vi "Download Waveform.vi"(0 "RFSG handle":refnum<k15>, 5 "Waveform In":T1={"Waveform Name"="Wfm", "Waveform"={"x0"=0.0, "dx"=0.0, "y"=[]}, "Signal Bandwidth (Hz)"=0.0, "PAPR (dB)"=0.0, "Burst Length (s)"=0.0, "Sample Rate"=0.0, "Burst Start Locations"=[], "Burst Stop Locations"=[], "Idle Duration Present?"=FALSE, "Runtime Scaling"=0.0, "Script"=""} {"Runtime Scaling" format="%#_6p"; "Sample Rate" format="%#_6p"; "Burst Length (s)" format="%#_6p"; "PAPR (dB)" format="%.2f"; "Signal Bandwidth (Hz)" format="%.2f"; "Waveform"."y" format="%.2f"; "Waveform"."dx" format="%^.2e"; "Waveform"."x0" format="%^.2e"}, 11 "error in (no error)":errorcluster) -> (4 "RFSG handle out":refnum<k15>, 15 "error out":errorcluster)   [LabVIEW 2016, in "SG.lvlib"]
uses:
  SG.lvlib
  Typedefs/Waveform.ctl
  <instrlib>/niRFSG/niRFSG.llb/niRFSG Write Arb Waveform (Complex Input SGL).vi
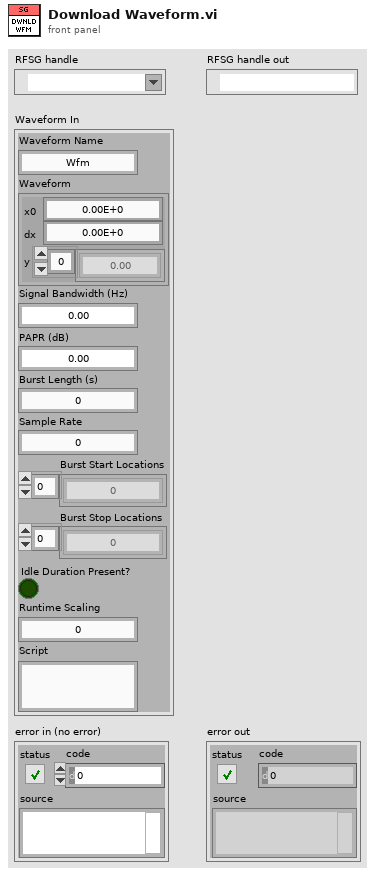
[diagram p1: front panel]
types:
  T1 = typedef "SG.lvlib/Waveform.ctl" = cluster{"Waveform Name":string, "Waveform":cluster{"x0":dbl, "dx":dbl, "y":csg[]}, "Signal Bandwidth (Hz)":dbl, "PAPR (dB)":dbl, "Burst Length (s)":dbl, "Sample Rate":dbl, "Burst Start Locations":i32[], "Burst Stop Locations":i32[], "Idle Duration Present?":bool, "Runtime Scaling":dbl, "Script":string}
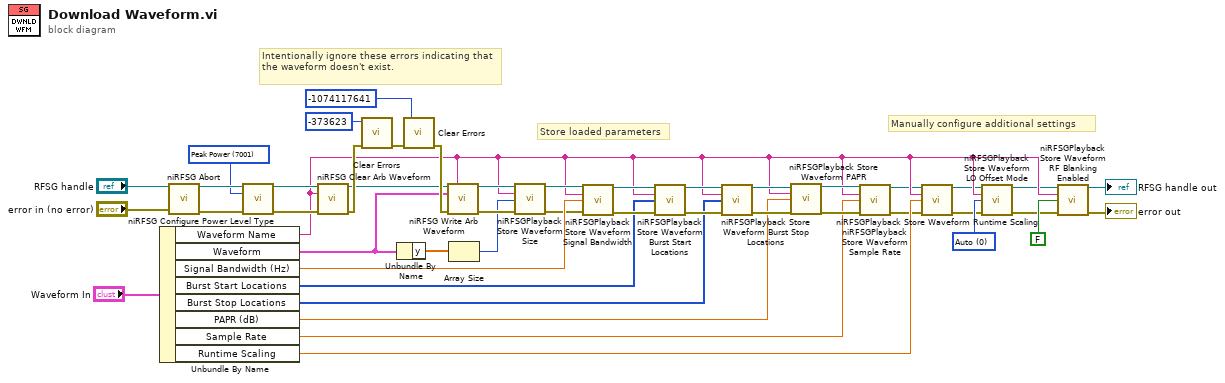
[diagram p0: block diagram]
diagram:
  w16 = 7001 items=["Average Power"=7000, "Peak Power"=7001] ("power level type")
  w32 = 0 items=["Auto", "No Offset", "Disabled"] ("LO offset mode")
  # "Manually configure additional settings"
  # "Store loaded parameters"
  # "Intentionally ignore these errors indicating that the waveform doesn't exist."
  n1 = Unbundle By Name("Waveform In") -> ("Waveform Name"=w7:string, "Waveform"=w10:cluster{"x0":dbl, "dx":dbl, "y":csg[]}, "Signal Bandwidth (Hz)"=w30:dbl, "Burst Start Locations"=w27:i32[], "Burst Stop Locations"=w24:i32[], "PAPR (dB)"=w23:dbl, "Sample Rate"=w19:dbl, "Runtime Scaling"=w14:dbl)
  n2 = call <instrlib>:"niRFSG Abort.vi"("instrument handle"="RFSG handle", "error in"="error in (no error)") -> ("instrument handle out"=w18:refnum<k15>, "error out"=w41:errorcluster)  [unwired: 12 in]
  n3 = call <instrlib>:"niRFSG Configure Power Level Type.vi"("instrument handle"=w18, "power level type"=w16, "error in"=w41) -> ("instrument handle out"=w17:refnum<k15>, "error out"=w36:errorcluster)  [unwired: 11 in]
  n4 = call <instrlib>:"niRFSG Clear Arb Waveform.vi"("instrument handle"=w17, "name"=w7, "error in"=w36) -> ("instrument handle out"=w31:refnum<k15>, "error out"=w40:errorcluster)  [unwired: 11 in]
  n5 = call <vilib>:"Clear Errors.vi"("error in (no error)"=w40, "specific error code to clear (0: all)"=-373623) -> ("error out"=w44:errorcluster)  [unwired: 4 in, 1 out]
  n6 = Unbundle By Name(w10) -> ("y"=w9:csg[])
  n7 = call <vilib>:"Clear Errors.vi"("error in (no error)"=w44, "specific error code to clear (0: all)"=-1074117641) -> ("error out"=w43:errorcluster)  [unwired: 4 in, 1 out]
  n8 = call-poly <instrlib>:"niRFSG Write Arb Waveform.vi"("instrument handle"=w31, "name"=w7, "IQ waveform"=w10, "error in"=w43) -> ("instrument handle out"=w12:refnum<k15>, "error out"=w15:errorcluster)  [unwired: 10 in]
  n9 = Array Size(array=w9) -> (size(s)=w8:i32)
  n10 = call <instrlib>:"niRFSGPlayback Store Waveform Size.vi"("instrument handle in"=w12, "waveform name"=w7, "waveform size"=w8, "error in"=w15) -> ("instrument handle out"=w11:refnum<k15>, "error out"=w13:errorcluster)  [unwired: 10 in]
  n11 = call <instrlib>:"niRFSGPlayback Store Waveform Signal Bandwidth.vi"("instrument handle in"=w11, "waveform name"=w7, "signal bandwidth"=w30, "error in"=w13) -> ("instrument handle out"=w28:refnum<k15>, "error out"=w42:errorcluster)  [unwired: 10 in]
  n12 = call <instrlib>:"niRFSGPlayback Store Waveform Burst Start Locations.vi"("instrument handle in"=w28, "waveform name"=w7, "burst start locations"=w27, "error in"=w42) -> ("instrument handle out"=w26:refnum<k15>, "error out"=w39:errorcluster)  [unwired: 10 in]
  n13 = call <instrlib>:"niRFSGPlayback Store Waveform Burst Stop Locations.vi"("instrument handle in"=w26, "waveform name"=w7, "burst stop locations"=w24, "error in"=w39) -> ("instrument handle out"=w25:refnum<k15>, "error out"=w38:errorcluster)  [unwired: 10 in]
  n14 = call <instrlib>:"niRFSGPlayback Store Waveform PAPR.vi"("instrument handle in"=w25, "waveform name"=w7, "PAPR"=w23, "error in"=w38) -> ("instrument handle out"=w20:refnum<k15>, "error out"=w45:errorcluster)  [unwired: 10 in]
  n15 = call <instrlib>:"niRFSGPlayback Store Waveform Sample Rate.vi"("instrument handle in"=w20, "waveform name"=w7, "sample rate"=w19, "error in"=w45) -> ("instrument handle out"=w4:refnum<k15>, "error out"=w3:errorcluster)  [unwired: 10 in]
  n16 = call <instrlib>:"niRFSGPlayback Store Waveform Runtime Scaling.vi"("instrument handle in"=w4, "waveform name"=w7, "runtime scaling"=w14, "error in"=w3) -> ("instrument handle out"=w6:refnum<k15>, "error out"=w5:errorcluster)  [unwired: 10 in]
  n17 = call <instrlib>:"niRFSGPlayback Store Waveform LO Offset Mode.vi"("instrument handle in"=w6, "waveform name"=w7, "LO offset mode"=w32, "error in"=w5) -> ("instrument handle out"=w2:refnum<k15>, "error out"=w1:errorcluster)  [unwired: 10 in]
  n18 = call <instrlib>:"niRFSGPlayback Store Waveform RF Blanking Enabled.vi"("instrument handle in"=w2, "waveform name"=w7, "RF blanking enabled"=FALSE, "error in"=w1) -> ("instrument handle out"=→"RFSG handle out":refnum<k15>, "error out"=→"error out":errorcluster)  [unwired: 10 in]
